vi "FGV Plot ausschalten.vi"() -> ()   [LabVIEW 2015]
uses:
  Aktion Plot.ctl
panel:
  in  "Aktiviert":bool
  in  "Aktion":T1
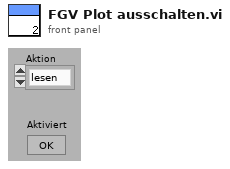
[diagram p1: front panel]
types:
  T1 = typedef "Aktion Plot.ctl" = enum16{"lesen", "schreiben", "init"}
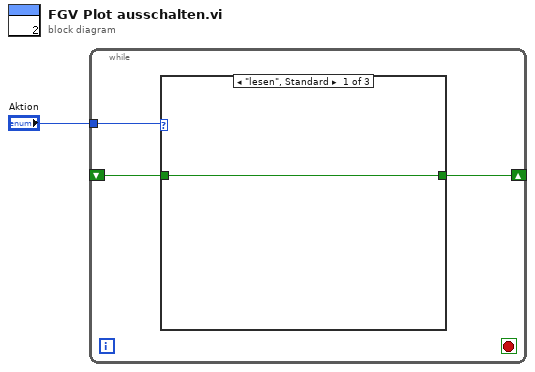
[diagram p0: block diagram]
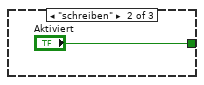
[diagram p2: hidden frame]
diagram:
  n1 = while {
    tunnel: "Aktion" -> [w4]
    shift-right: [w3] -> _
    shift-left: _ -> [w2]
    stop <- _ stop-if-true
    n2 = case shown="\"lesen\", Standard" w4 {
      tunnel: [w5 "Aktiviert" w7] -> w3
      tunnel: w2 -> [w5 _ w7]
      frame "lesen", Default {
      }
      frame "schreiben" {
      }
      frame "init" {
      }
    }
  }
